vi "remove_background.vi"(0 "Array in":cdb[][](array[numeric])) -> (2 "Array out":cdb[][](array[numeric]))   [LabVIEW 2013]
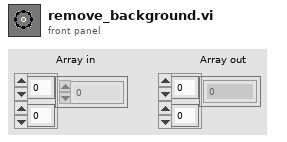
[diagram p1: front panel]
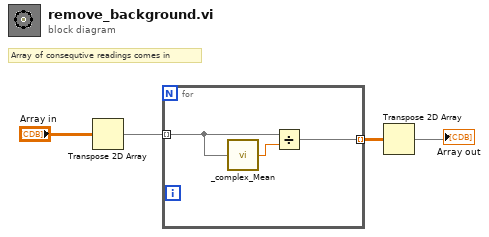
[diagram p0: block diagram]
diagram:
  # "Array of consequtive readings comes in"
  n1 = Transpose 2D Array(2D array="Array in") -> (transposed array=w1:cdb[][])
  n2 = for "Remove background noise" {
    tunnel: w1 -> [w7] mode=indexing
    tunnel: [w6] -> w2 mode=indexing
    n3 = call "_complex_Mean.vi"("Zin"=w7) -> ("Numeric"=w5:cdb)
    n4 = Divide(x=w7, y=w5) -> (x/y=w6:cdb[])
  }
  n5 = Transpose 2D Array(2D array=w2) -> (transposed array=→"Array out":cdb[][])
